vi "Bundle.vi"(8 "error in (no error)":errorcluster, 9 "Close reference after insertion(F)":bool, 10 "Sub Panel":refnum<vi>, 11 "Sub Panel Insertion Msg in":refnum<class "Sub Panel Insertion Msg.lvclass">) -> (0 "error out":errorcluster, 3 "Sub Panel Insertion Msg out":refnum<class "Sub Panel Insertion Msg.lvclass">)   [LabVIEW 2020, in "Msg.lvlib" / "Sub Panel Insertion Msg.lvclass"]
doc: "Write a sub panel reference and whether the reference should be closed after the VI insertion or not, to the Sub Panel Insertion Msg private data."
uses:
  Sub Panel Insertion Msg.lvclass
  Sub Panel Insertion Msg.lvclass/Sub Panel Insertion Msg.ctl
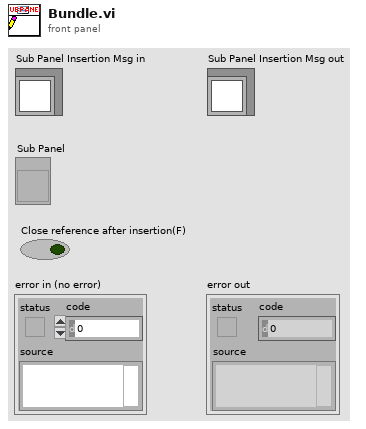
[diagram p1: front panel]
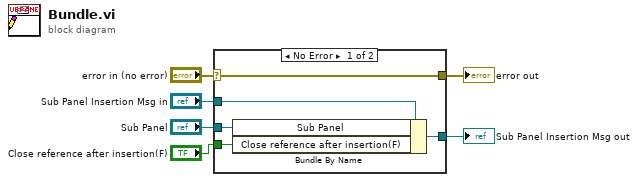
[diagram p0: block diagram]
diagram:
  n1 = case shown="No Error" "error in (no error)" {
    selector: "error in (no error)" -> [w11 w12]
    tunnel: [w11 w12] -> w5
    tunnel: [w9 w13] -> w3
    tunnel: "Sub Panel Insertion Msg in" -> [w10 w13]
    tunnel: "Sub Panel" -> [w8 _]
    tunnel: "Close reference after insertion(F)" -> [w7 _]
    frame No Error {
      n2 = Bundle By Name(cluster=w10, "Sub Panel"=w8, "Close reference after insertion(F)"=w7) -> (w9:refnum<class "Sub Panel Insertion Msg.lvclass">)
    }
    frame Error {
    }
  }
  "error out" <- w5
  "Sub Panel Insertion Msg out" <- w3
